vi "Map License Type.vi"(10 "TS License Type":T1) -> (2 "license":i32)   [LabVIEW 2020, in "TSS.lvlib" / "Engine.lvclass"]
uses:
  Engine.lvclass
  TS License Type.ctl
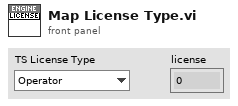
[diagram p1: front panel]
types:
  T1 = typedef "TSS.lvlib/Engine.lvclass/TS License Type.ctl" = enum16{"Operator", "CustomEditor", "SequenceEditor"}
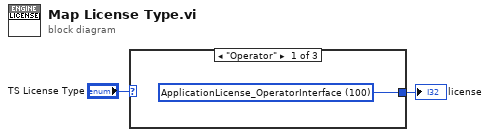
[diagram p0: block diagram]
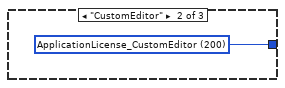
[diagram p2: hidden frame]
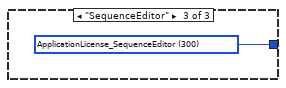
[diagram p3: hidden frame]
diagram:
  n1 = case shown="\"Operator\"" "TS License Type" {
    tunnel: [w3 w4 w5] -> w1
    frame "Operator" {
      w3 = 100 items=["ApplicationLicense_Unspecified"=0, "ApplicationLicense_OperatorInterface"=100, "ApplicationLicense_CustomEditor"=200, "ApplicationLicense_SequenceEditor"=300] ("license")
    }
    frame "CustomEditor" {
      w4 = 200 items=["ApplicationLicense_Unspecified"=0, "ApplicationLicense_OperatorInterface"=100, "ApplicationLicense_CustomEditor"=200, "ApplicationLicense_SequenceEditor"=300] ("license")
    }
    frame "SequenceEditor" {
      w5 = 300 items=["ApplicationLicense_Unspecified"=0, "ApplicationLicense_OperatorInterface"=100, "ApplicationLicense_CustomEditor"=200, "ApplicationLicense_SequenceEditor"=300] ("license")
    }
  }
  "license" <- w1
